vi "find qubit resonance.vi"() -> ()   [LabVIEW 2021]
uses:
  <vilib>/Utility/file.llb/Write Delimited Spreadsheet (DBL).vi
panel:
  in  "Sample Name":string
  in  "base path":path=path "C:/Users/dvh-collab-user/Desktop/20221122 Robert qubit"
  out "Plot 2":cluster{"output array":dbl[], dbl[]}[](graph)
  in  "Stop Button":bool
  out "Plot":cluster{"output array":dbl[], dbl[]}[](graph)
  in  "Tab Control":enum32{"LO", "VNA", "Error"}(tab)
  in  "End Fre GHz":dbl=4.522 format="%.10f"
  in  "Step Fre MHz":dbl=0.01 format="%.10f"
  in  "LO Chan":u16(ring)=1 items=["Channel 2"=2, "Channel 1"=1]
  in  "Start Fre GHz":dbl=4.516 format="%.10f"
  in  "Power dBm":dbl format="%#.3f"
  in  "LO Init":bool
  in  "Delay Time s":dbl=0.1
  in  "VNA address":string="P9374A"
  in  "Avg number":i32=100
  in  "Frequency Hz":dbl=6.0237 caption="Cavity Fre GHz" format="%#_6f"
  in  "Power dBm 2":dbl=-20.0 caption="VNA Power dBm"
  out "error out":errorcluster
  # "This VI apply LO RF and sweep the frequency, while measure S21 at fixed frequency point from NA"
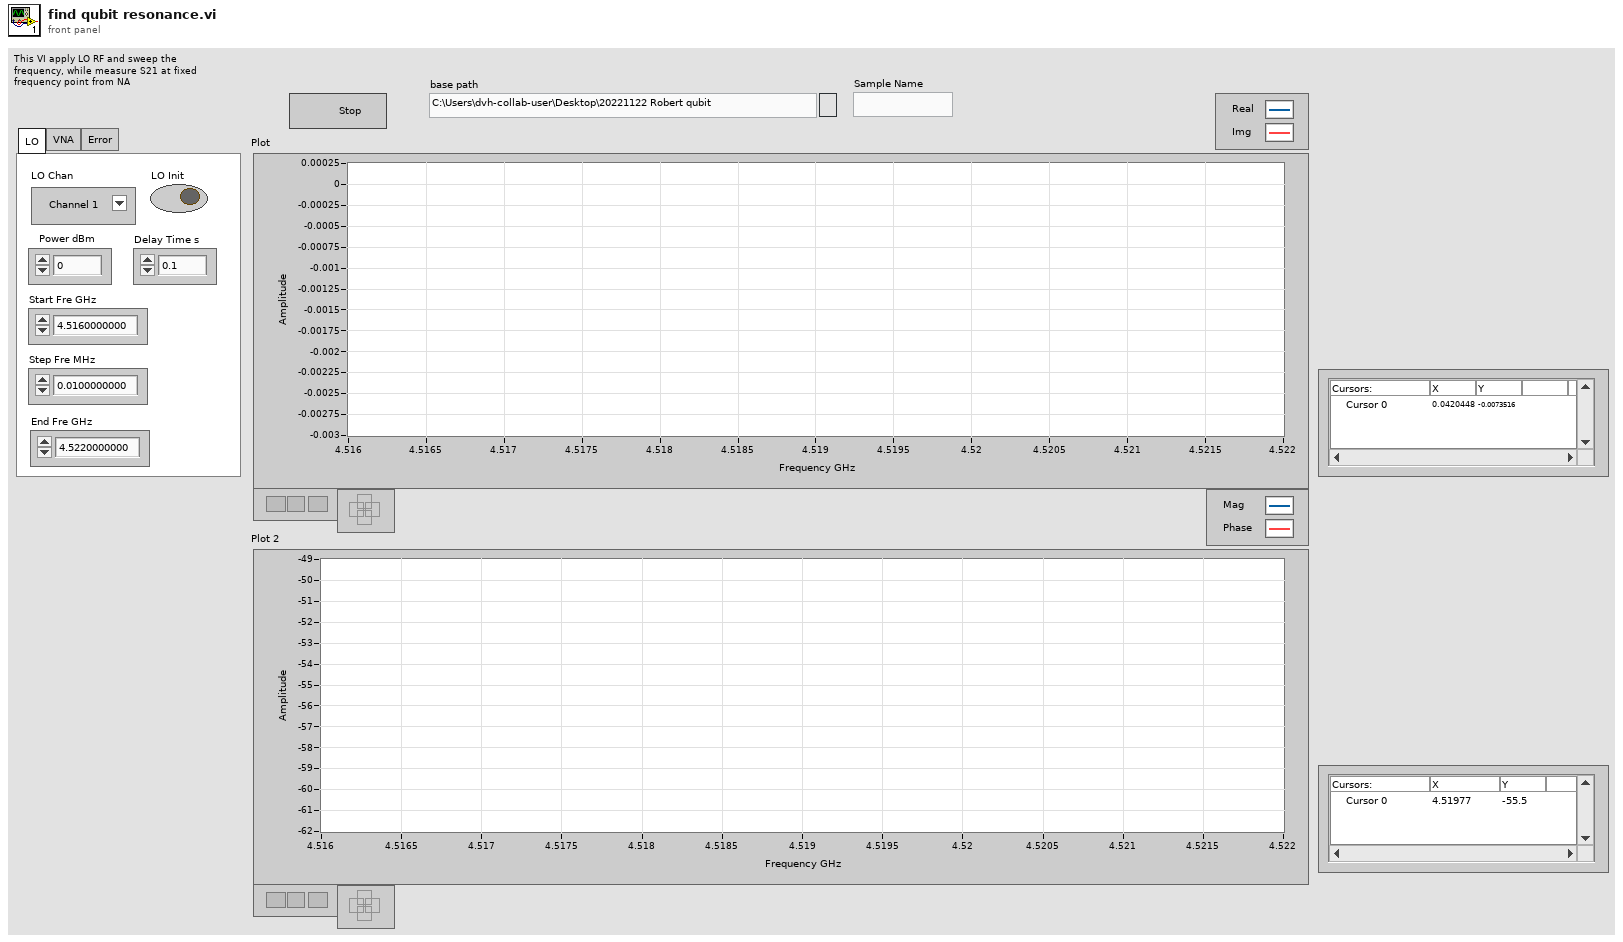
[diagram p1: front panel]
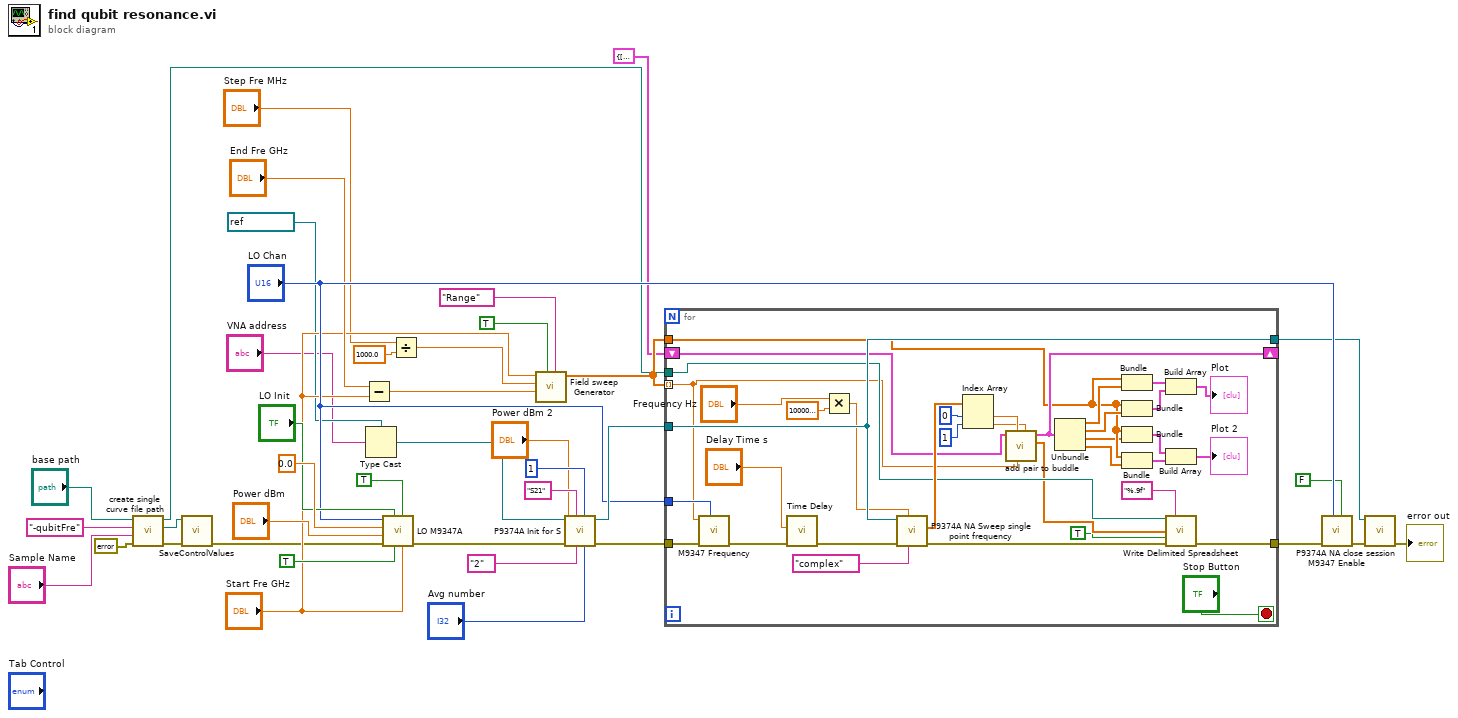
[diagram p0: block diagram]
diagram:
  n1 = call "create single curve file path.vi"("base path"="base path", "Measurement Name"="-qubitFre", "Sample Name"="Sample Name", "error in (no error)"=errorcluster {"status"=FALSE, "code"=0, "source"=""}) -> ("data path"=w8:path, "para path"=w10:path, "error out"=w11:errorcluster)  [unwired: 4 in]
  n2 = call "SaveControlValues.vi"("XML File Path"=w10, "error in (no error)"=w11) -> ("error out"=w9:errorcluster)  [unwired: 8 in]
  n3 = Subtract(x="End Fre GHz", y="Start Fre GHz") -> (x-y=w18:dbl)
  n4 = Type Cast(type=refnum<k15> "P9374A" ("resource name"), x="VNA address") -> (*(type *) &x=w5:refnum<k15>)
  n5 = call "LO M9347A.vi"("Frequency GHz"="Start Fre GHz", "Exec"=TRUE, "Enable"=TRUE, "Init"="LO Init", "error in (no error)"=w9, "Power dBm"="Power dBm", "Phase degree"=0.0, "Chan"="LO Chan") -> ("error out"=w33:errorcluster)  [unwired: 3 in]
  n6 = Divide(x="Step Fre MHz", y=1000.0) -> (x/y=w3:dbl)
  n7 = call "Field sweep Generator.vi"("Ramp type"="Range", "Ramp up first T"=TRUE, "Field Radius"=w18, "Field step"=w3, "Field Origin"="Start Fre GHz") -> ("output array"=w17:dbl[])  [unwired: 6 in]
  n8 = call "P9374A Init for S.vi"("Avg number"="Avg number", "points"=1, "Port source to be off"="2", "ChannelParameter"="S21", "error in (no error)"=w33, "Power dBm"="Power dBm 2", "resource name"=w5) -> ("error out"=w28:errorcluster, "instrument handle out"=w27:refnum<k15>)  [unwired: 3 in]
  n9 = for {
    tunnel: w17 -> [w46] mode=indexing
    tunnel: "LO Chan" -> [w76]
    tunnel: w28 -> [w75]
    tunnel: w27 -> [w72]
    tunnel: [w41] -> w26
    tunnel: [w72] -> w22
    shift-right: [w64] -> _
    shift-left: cluster{dbl[], dbl[], dbl[], dbl[]} {[], [], [], []} ("output") -> [w67]
    tunnel: w17 -> [w54]
    tunnel: w8 -> [w48]
    stop <- "Stop Button" stop-if-true
    n10 = call "M9347 Frequency.vi"("Chan"=w76, "error in (no error)"=w75, "Frequency GHz"=w46) -> ("error out"=w74:errorcluster)  [unwired: 8 in]
    n11 = call "Time Delay"("error in (no error)"=w74, "Delay Time (s)"="Delay Time s") -> ("error out"=w73:errorcluster)  [unwired: 9 in]
    n12 = Multiply(x="Frequency Hz", y=1000000000.0) -> (x*y=w47:dbl)
    n13 = call "P9374A NA Sweep single point frequency.vi"("Data type"="complex", "Frequency Hz"=w47, "error in (no error)"=w73, "instrument handle"=w72) -> ("error out"=w44:errorcluster, "Val"=w71:dbl[])  [unwired: 5 in, 1 out]
    n14 = Index Array(array=w71, index #1=0 ("index"), index #2=1 ("index")) -> (element #1=w66:dbl, element #2=w65:dbl)
    n15 = call "add pair to buddle.vi"("y"=w65, "fre"=w46, "x"=w66, "Input"=w67) -> ("array"=w45:dbl[], "output"=w64:cluster{dbl[], dbl[], dbl[], dbl[]})  [unwired: 6 in]
    n16 = Unbundle(w64) -> (w63:dbl[], w62:dbl[], w53:dbl[], w52:dbl[])
    n17 = Bundle("output array"=w54, w63) -> (w61:cluster{"output array":dbl[], dbl[]})  [unwired: 1 in]
    n18 = Bundle("output array"=w54, w62) -> (w60:cluster{"output array":dbl[], dbl[]})  [unwired: 1 in]
    n19 = Bundle("output array"=w54, w53) -> (w51:cluster{"output array":dbl[], dbl[]})  [unwired: 1 in]
    n20 = Bundle("output array"=w54, w52) -> (w50:cluster{"output array":dbl[], dbl[]})  [unwired: 1 in]
    n21 = Build Array(w61, w60) -> (→"Plot":cluster{"output array":dbl[], dbl[]}[])
    n22 = Build Array(w51, w50) -> (→"Plot 2":cluster{"output array":dbl[], dbl[]}[])
    n23 = call-poly <vilib>:"Write Delimited Spreadsheet.vi"("file path (dialog if empty)"=w48, "format (%.3f)"="%.9f", "1D data"=w45, "append to file? (new file:F)"=TRUE, "error in (no error)"=w44) -> ("error out"=w41:errorcluster)  [unwired: 9 in, 1 out]
  }
  n24 = call "M9347 Enable.vi"("Enable"=FALSE, "Chan"="LO Chan", "error in (no error)"=w26) -> ("error out"=w23:errorcluster)  [unwired: 8 in]
  n25 = call "P9374A NA close session.vi"("error in (no error)"=w23, "instrument handle"=w22) -> ("error out"=→"error out":errorcluster)  [unwired: 9 in]
